vi "rad_Discover Bitfiles In Image Zip.vi"(8 "error in (no error)":errorcluster, 11 "Image Path":path) -> (0 "error out":errorcluster, 2 "Bitfiles Found":string[](array[string]), 3 "Image Path Out":path)   [LabVIEW 2013]
uses:
  <vilib>/zip/NI_Unzip.lvlib
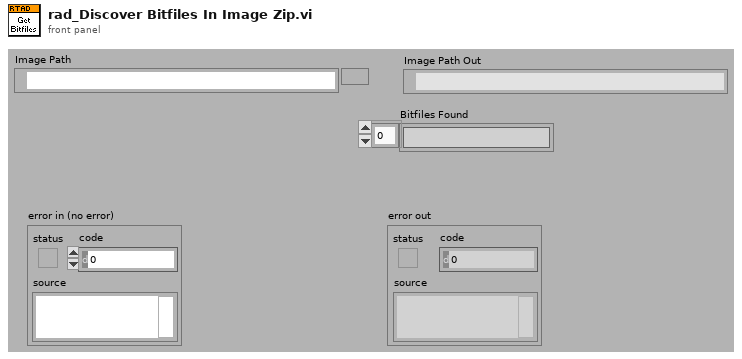
[diagram p1: front panel]
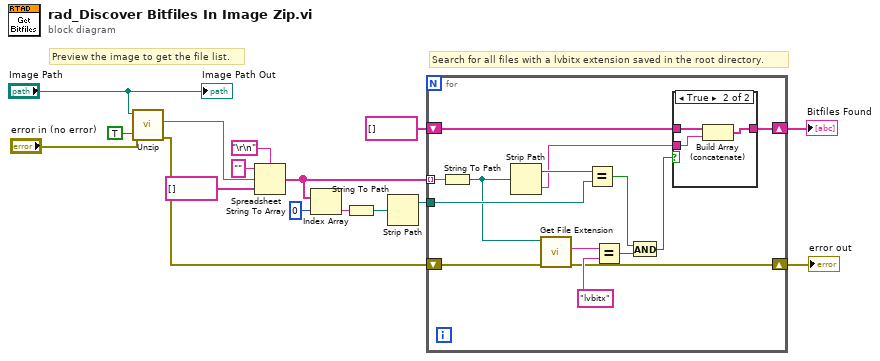
[diagram p0: block diagram]
diagram:
  # "Search for all files with a lvbitx extension saved in the root directory."
  # "Preview the image to get the file list."
  n1 = call <vilib>:"Unzip.vi"("error in (no error)"="error in (no error)", "Preview only?"=TRUE, "Zip file"="Image Path") -> ("error out"=w4:errorcluster, "Preview"=w14:string)  [unwired: 6 in, 1 out]
  n2 = Spreadsheet String To Array(delimiter (Tab)="\r\n", format string="", spreadsheet string=w14, array type (2D Dbl)=string[] []) -> (array=w12:string[])
  n3 = Index Array(array=w12, index=0) -> (element=w11:string)
  n4 = String To Path(string=w11) -> (path=w9:path)
  n5 = Strip Path(path=w9) -> (stripped path=w8:path)  [unwired: 1 out]
  n6 = for {
    tunnel: w12 -> [w26] mode=indexing
    tunnel: w8 -> [w24]
    shift-right: [w21] -> w6
    shift-left: string[] [] -> [w20]
    shift-right: [w17] -> w1
    shift-left: w4 -> [w18]
    n7 = String To Path(string=w26) -> (path=w22:path)
    n8 = Strip Path(path=w22) -> (stripped path=w25:path, name=w19:string)
    n9 = call <vilib>:"Get File Extension.vi"("error in (no error)"=w18, "file"=w22) -> ("error out"=w17:errorcluster, "lowercase file extension"=w30:string)  [unwired: 6 in, 2 out]
    n10 = Equal?(x=w25, y=w24) -> (x = y?=w23:bool)
    n11 = Equal?(x=w30, y="lvbitx") -> (x = y?=w28:bool)
    n12 = And(x=w23, y=w28) -> (x .and. y?=w27:bool)
    n13 = case shown="True" w27 {
      tunnel: [w31 w34] -> w21
      tunnel: w20 -> [w31 w33]
      tunnel: w19 -> [_ w32]
      frame False {
      }
      frame True {
        n14 = Build Array (concatenate)(w33, w32) -> (w34:string[])
      }
    }
  }
  "error out" <- w1
  "Bitfiles Found" <- w6
  "Image Path Out" <- "Image Path"
